vi "Get Max Block Count.vi"(8 "error in (no error)":errorcluster, 10 "previous block count (0)":u64, 11 "Transfer Group in":refnum<class "Transfer Group.lvclass">) -> (0 "error out":errorcluster, 2 "largest block count":u64, 3 "Transfer Group out":refnum<class "Transfer Group.lvclass">)   [LabVIEW 2017, in "Data Sharing Framework Core.lvlib" / "Data Sharing Framework Engine.lvlib" / "Transfer Group.lvclass"]
uses:
  Transfer Group.lvclass
  Transfer Group.lvclass/Transfer Group.ctl
  Transfer/Transfer.lvclass
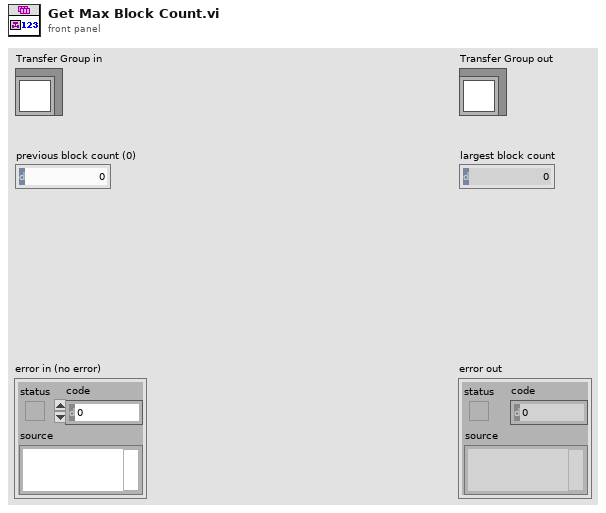
[diagram p1: front panel]
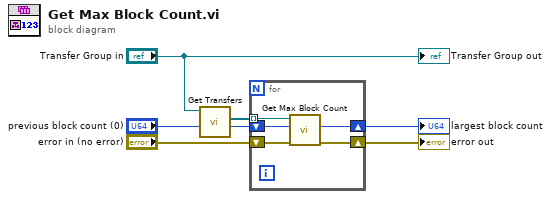
[diagram p0: block diagram]
diagram:
  n1 = call "Get Transfers.vi"("Transfer Group in"="Transfer Group in") -> ("Transfers"=w6:refnum<class "Transfer.lvclass">[])  [unwired: 9 in, 1 out]
  n2 = for {
    tunnel: w6 -> [w11] mode=indexing
    shift-right: [w8] -> w5
    shift-left: "previous block count (0)" -> [w7]
    shift-right: [w10] -> w2
    shift-left: "error in (no error)" -> [w9]
    n3 = call "Get Max Block Count.vi"("error in (no error)"=w9, "previous block count (0)"=w7, "Transfer in"=w11) -> ("error out"=w10:errorcluster, "largest block count"=w8:u64)  [unwired: 6 in, 1 out]
  }
  "error out" <- w2
  "largest block count" <- w5
  "Transfer Group out" <- "Transfer Group in"
